vi "Compare_Timestamps.vi"(9 "Time stamp 2":T2, 10 "Time stamp 1":T2) -> (2 "Comparison result":T1)   [LabVIEW 2013]
uses:
  Controls/GPS_Timestamp.ctl
  Controls/Comparison_Result.ctl
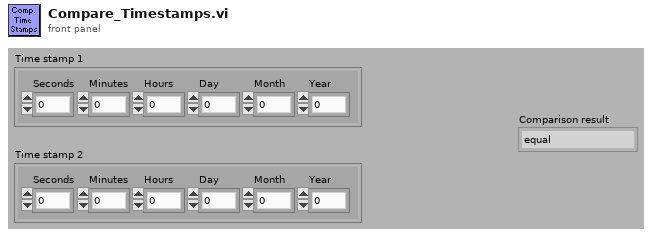
[diagram p1: front panel]
types:
  T1 = typedef "Comparison_Result.ctl" = enum16{"equal", "1 < 2", "1 > 2", "error in 1", "error in 2", "error in both"}
  T2 = typedef "GPS_Timestamp.ctl" = cluster{"Seconds":u8, "Minutes":u8, "Hours":u8, "Day":u8, "Month":u8, "Year":u16}
  T3 = cluster{"second":i32, "minute":i32, "hour":i32, "day of month":i32, "month":i32, "year":i32, "day of week":i32, "day of year":i32, "is DST":i32}
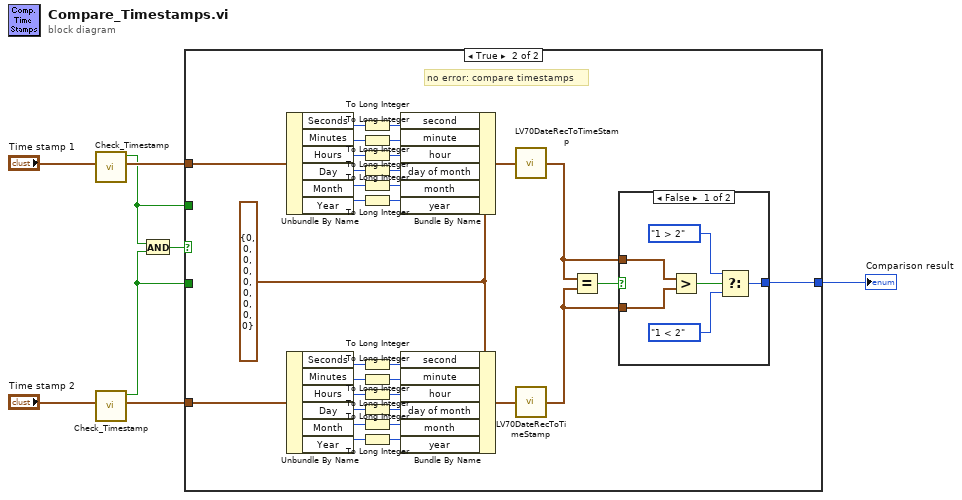
[diagram p0: block diagram]
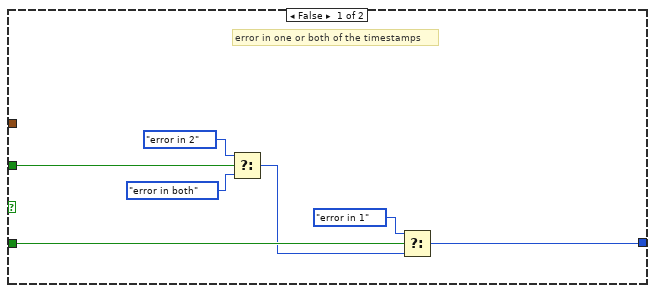
[diagram p2: hidden frame]
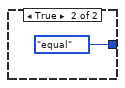
[diagram p3: hidden frame]
diagram:
  n1 = call "Check_Timestamp.vi"("Time stamp in"="Time stamp 1") -> ("Time stamp out"=w5:T2, "Result"=w4:bool)  [unwired: 9 out]
  n2 = call "Check_Timestamp.vi"("Time stamp in"="Time stamp 2") -> ("Time stamp out"=w2:T2, "Result"=w1:bool)  [unwired: 9 out]
  n3 = And(x=w4, y=w1) -> (x .and. y?=w7:bool)
  n4 = case shown="True" w7 {
    tunnel: w5 -> [_ w35]
    tunnel: w2 -> [_ w21]
    tunnel: [w15 w19] -> w8
    tunnel: w4 -> [w10 _]
    tunnel: w1 -> [w13 _]
    frame False {
      # "error in one or both of the timestamps"
      # "there is an error in one of the timestamps"
      n5 = Select(t=Comparison_Result."error in 2" ("Comparison result"), s=w10, f=Comparison_Result."error in both") -> (s? t:f=w11:T1)
      n6 = Select(t=Comparison_Result."error in 1" ("Comparison result"), s=w13, f=w11) -> (s? t:f=w15:T1)
    }
    frame True {
      w20 = T3 {"second"=0, "minute"=0, "hour"=0, "day of month"=0, "month"=0, "year"=0, "day of week"=0, "day of year"=0, "is DST"=0} ("date time rec")
      # "no error: compare timestamps"
      n7 = Unbundle By Name(w35) -> ("Seconds"=w48:u8, "Minutes"=w47:u8, "Hours"=w46:u8, "Day"=w45:u8, "Month"=w44:u8, "Year"=w43:u16)
      n8 = Unbundle By Name(w21) -> ("Seconds"=w34:u8, "Minutes"=w33:u8, "Hours"=w32:u8, "Day"=w31:u8, "Month"=w30:u8, "Year"=w29:u16)
      n9 = To Long Integer(number=w48) -> (32bit integer=w42:i32)
      n10 = To Long Integer(number=w47) -> (32bit integer=w41:i32)
      n11 = To Long Integer(number=w46) -> (32bit integer=w40:i32)
      n12 = To Long Integer(number=w45) -> (32bit integer=w39:i32)
      n13 = To Long Integer(number=w44) -> (32bit integer=w38:i32)
      n14 = To Long Integer(number=w43) -> (32bit integer=w37:i32)
      n15 = To Long Integer(number=w34) -> (32bit integer=w28:i32)
      n16 = To Long Integer(number=w33) -> (32bit integer=w27:i32)
      n17 = To Long Integer(number=w32) -> (32bit integer=w26:i32)
      n18 = To Long Integer(number=w31) -> (32bit integer=w25:i32)
      n19 = To Long Integer(number=w30) -> (32bit integer=w24:i32)
      n20 = To Long Integer(number=w29) -> (32bit integer=w23:i32)
      n21 = Bundle By Name(cluster=w20, "second"=w42, "minute"=w41, "hour"=w40, "day of month"=w39, "month"=w38, "year"=w37) -> (w36:T3)
      n22 = Bundle By Name(cluster=w20, "second"=w28, "minute"=w27, "hour"=w26, "day of month"=w25, "month"=w24, "year"=w23) -> (w22:T3)
      n23 = call <vilib>:"LV70DateRecToTimeStamp.vi"("date time rec"=w36) -> ("Time Stamp"=w17:timestamp)
      n24 = call <vilib>:"LV70DateRecToTimeStamp.vi"("date time rec"=w22) -> ("Time Stamp"=w16:timestamp)
      n25 = Equal?(x=w17, y=w16) -> (x = y?=w18:bool)
      n26 = case shown="False" w18 {
        tunnel: [w49 Comparison_Result."equal" ("Comparison result")] -> w19
        tunnel: w17 -> [w54 _]
        tunnel: w16 -> [w53 _]
        frame False {
          n27 = Greater?(x=w54, y=w53) -> (0:w52:bool)
          n28 = Select(t=Comparison_Result."1 > 2" ("Comparison result"), s=w52, f=Comparison_Result."1 < 2" ("Comparison result")) -> (s? t:f=w49:T1)
        }
        frame True {
        }
      }
    }
  }
  "Comparison result" <- w8
